vi "Wavefrom Subsets from Cursors.vi"(8 "Error In":errorcluster, 9 "Waveforms In":waveform(dbl)[][](array[waveform]), 11 "Waveform Graph":refnum<vi>) -> (0 "Error Out":errorcluster, 1 "Waveform Subsets":waveform(dbl)[][](array[waveform]))   [LabVIEW 2017]
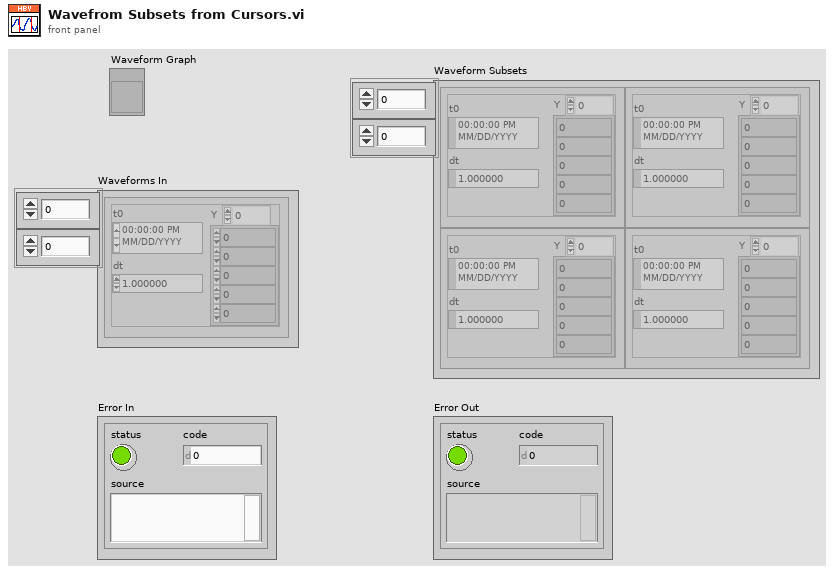
[diagram p1: front panel]
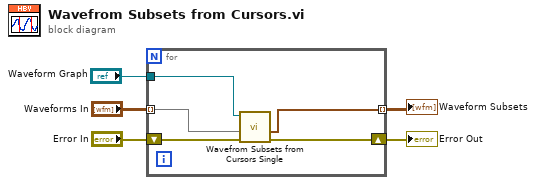
[diagram p0: block diagram]
diagram:
  n1 = for {
    shift-right: [w10] -> w5
    shift-left: "Error In" -> [w9]
    tunnel: [w6] -> w1 mode=indexing
    tunnel: "Waveforms In" -> [w8] mode=indexing
    tunnel: "Waveform Graph" -> [w7]
    n2 = call "Wavefrom Subsets from Cursors Single.vi"("Error In"=w9, "Waveforms In"=w8, "Waveform Graph"=w7) -> ("Error Out"=w10:errorcluster, "Waveform Subsets"=w6:waveform(dbl)[])  [unwired: 7 in]
  }
  "Error Out" <- w5
  "Waveform Subsets" <- w1
